vi "test Encoding Error Conditions.vi"(8 "error in":errorcluster, 11 "TestCase in":refnum<class "Encoding and Decoding.lvclass">) -> (0 "error out":errorcluster, 3 "TestCase out":refnum<class "Encoding and Decoding.lvclass">)   [LabVIEW 2020, in "Encoding and Decoding.lvclass"]
uses:
  Encoding and Decoding.lvclass
  Protocol/Implementations/ARINC429/Parameter Definition.ctl
  Encoding and Decoding/Encoding.ctl
  Protocol/Implementations/ARINC429/ARINC429-32bit/32-bit Word.lvclass/32-bit Word.ctl
  4413749d-09be-4b2c-9fd8-42957a21c6ba.vi
  Shared/Encode Parameter and Update Word (32-bit).vi/1445f95d-237d-4fc6-96b9-8992d347f513.vi
  Shared/Encode Parameter and Update Word (32-bit).vi/6b8853f0-8e5d-49e3-9391-4d3f8e5314b0.vi
  Shared/Encode Parameter and Update Word (32-bit).vi/2babc4f4-546e-4d35-846d-a4a1fbac0249.vi
  4413749d-09be-4b2c-9fd8-42957a21c6ba.vi/1980749b-e417-4a21-943a-7c30016504b0.vi
  4413749d-09be-4b2c-9fd8-42957a21c6ba.vi/1f3c3557-5c17-491c-9e18-ef0b55369bc3.vi
  Shared/Encode Parameter and Update Word (32-bit).vi/1445f95d-237d-4fc6-96b9-8992d347f513.vi/22abf0d2-70bd-4b51-a478-b97a2704f7df.vi
  Shared/Encode Parameter and Update Word (32-bit).vi/1445f95d-237d-4fc6-96b9-8992d347f513.vi/c253b733-33bf-43c6-b07a-ea22f5c7a6f3.vi
  Shared/Encode Parameter and Update Word (32-bit).vi/1445f95d-237d-4fc6-96b9-8992d347f513.vi/9377bb8f-44b5-4a8f-87f1-966fd5a9edcc.vi
  Shared/Encode Parameter and Update Word (32-bit).vi/6b8853f0-8e5d-49e3-9391-4d3f8e5314b0.vi/a54b505c-1216-4ef4-8378-3ceda9d188df.vi
  Shared/Encode Parameter and Update Word (32-bit).vi/6b8853f0-8e5d-49e3-9391-4d3f8e5314b0.vi/136dcdcb-2dd3-4a4d-a796-a8f7a3f8e1ac.vi
  4413749d-09be-4b2c-9fd8-42957a21c6ba.vi/1980749b-e417-4a21-943a-7c30016504b0.vi/16a2565b-3c16-407b-a626-9da2a3da432e.vi
  4413749d-09be-4b2c-9fd8-42957a21c6ba.vi/1f3c3557-5c17-491c-9e18-ef0b55369bc3.vi/0a001d06-2809-4638-8d0b-e017d2157007.vi
  Encoding and Decoding/BCD Decode Integer.vi
  Shared/Encode Parameter and Update Word (32-bit).vi/1445f95d-237d-4fc6-96b9-8992d347f513.vi/22abf0d2-70bd-4b51-a478-b97a2704f7df.vi/9d450a76-0fc9-4555-8e71-4c202274969f.vi
  Shared/Encode Parameter and Update Word (32-bit).vi/1445f95d-237d-4fc6-96b9-8992d347f513.vi/c253b733-33bf-43c6-b07a-ea22f5c7a6f3.vi/9d450a76-0fc9-4555-8e71-4c202274969f.vi
  Shared/Encode Parameter and Update Word (32-bit).vi/6b8853f0-8e5d-49e3-9391-4d3f8e5314b0.vi/a54b505c-1216-4ef4-8378-3ceda9d188df.vi/a7fcce85-1f75-4572-aeaa-ddfd463a7c5f.vi
  Encoding and Decoding/BCD Decode Integer.vi/9a65bfc0-0d77-4ef3-ab58-63df1e1caa90.vi
  Protocol/Implementations/ARINC429/ARINC429-32bit/32-bit Word.lvclass
  <vilib>/addons/_JKI Toolkits/VI Tester/TestCase.llb/TestCase.lvclass
  Encoding and Decoding/Encoding and Decoding.lvlib
  Protocol/Implementations/ARINC429/ARINC 429.lvclass
  C:/Program Files (x86)/National Instruments/LabVIEW 2020/vi.lib/addons/_JKI Toolkits/VI Tester/TestCase.llb/TestCase.lvclass
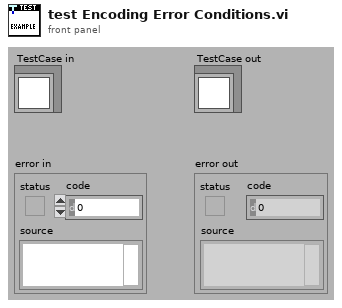
[diagram p1: front panel]
types:
  T1 = typedef "ARINC 429.lvclass/Parameter Definition.ctl" = cluster{"start index":i32, "size":i32, "encoding":T2, "signed":bool, "scale multiplier":dbl, "scale offset":dbl}
  T2 = typedef "Encoding and Decoding.lvlib/Encoding.ctl" = enum16{"BNR", "BCD", "Discrete"}
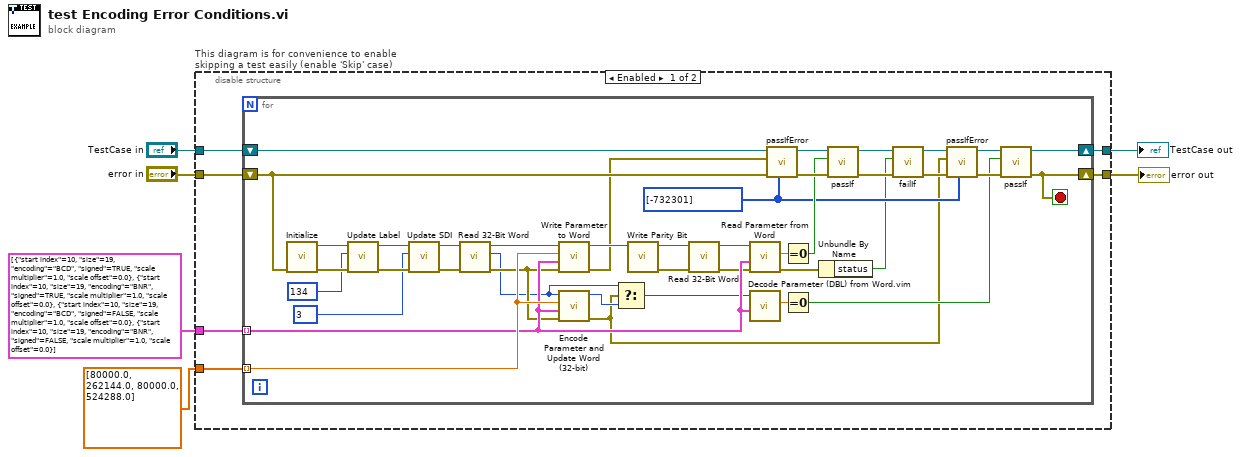
[diagram p0: block diagram]
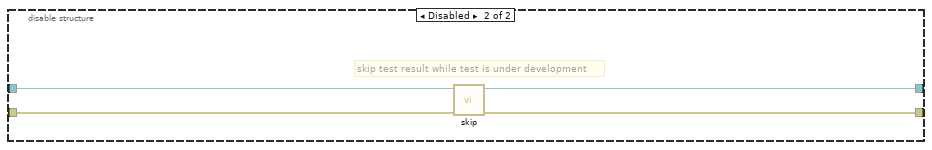
[diagram p2: hidden frame]
diagram:
  n1 = disable-structure "This diagram is for convenience to enable skipping a test easily (enable 'Skip' case)" shown="Enabled" {
    disable-tunnel: "TestCase in" -> [w12 w57]
    disable-tunnel: [w11 w55] -> w3
    disable-tunnel: [w10 w56] -> w5
    disable-tunnel: "error in" -> [w7 w54]
    disable-tunnel: T1[] [{"start index"=10, "size"=19, "encoding"=enum."BCD", "signed"=TRUE, "scale multiplier"=1.0, "scale offset"=0.0}, {"start index"=10, "size"=19, "encoding"=enum."BNR", "signed"=TRUE, "scale multiplier"=1.0, "scale offset"=0.0}, {"start index"=10, "size"=19, "encoding"=enum."BCD", "signed"=FALSE, "scale multiplier"=1.0, "scale offset"=0.0}, {"start index"=10, "size"=19, "encoding"=enum."BNR", "signed"=FALSE, "scale multiplier"=1.0, "scale offset"=0.0}] -> [w8 _]
    disable-tunnel: dbl[] [80000.0, 262144.0, 80000.0, 524288.0] -> [w9 _]
    frame Enabled {
      n2 = for {
        tunnel: w9 -> [w33] mode=indexing
        tunnel: w8 -> [w32] mode=indexing
        shift-right: [w34] -> w11
        shift-left: w12 -> [w40]
        shift-right: [w13] -> w10
        shift-left: w7 -> [w30]
        stop <- w13 stop-if-true
        w27 = i32[] [-732301] ("passing error codes (default = any error code)")
        n3 = call "Initialize.vi"("error in"=w30) -> ("error out"=w49:errorcluster, "ARINC 429 (32-bit word)"=w44:refnum<class "32-bit Word.lvclass">)  [unwired: 9 in]
        n4 = call-dynamic "Update Label.vi"("error in"=w49, "label value"=u8 134 ("label value 2"), "32-bit word in"=w44) -> ("error out"=w50:errorcluster, "32-bit word out"=w47:refnum<class "32-bit Word.lvclass">)  [unwired: 7 in]
        n5 = call-dynamic "Update SDI.vi"("error in"=w50, "SDI value"=u8 3 ("SDI value 2"), "32-bit Word in"=w47) -> ("error out"=w38:errorcluster, "32-bit Word out"=w39:refnum<class "32-bit Word.lvclass">)  [unwired: 7 in]
        n6 = call "Read 32-Bit Word.vi"("error in (no error)"=w38, "32-bit Word in"=w39) -> ("error out"=w26:errorcluster, "32-bit word"=w15:u32, "32-bit Word out"=w37:refnum<class "32-bit Word.lvclass">)  [unwired: 7 in]
        n7 = call-dynamic "Write Parameter to Word.vi"("error in"=w26, "parameter definition"=w32, "data"=w33, "32-bit Word in"=w37) -> ("error out"=w24:errorcluster, "32-bit Word out"=w52:refnum<class "32-bit Word.lvclass">)  [unwired: 6 in]
        n8 = call "Encode Parameter and Update Word (32-bit).vi"("error in"=w26, "parameter definition"=w32, "parameter value"=w33, "word in"=w15) -> ("error out"=w16:errorcluster, "word out"=w17:u32)  [unwired: 6 in]
        n9 = Select(t=w15, s=w16, f=w17) -> (s? t:f=w14:u32)
        n10 = call-dynamic "Write Parity Bit.vi"("32-bit word in"=w52) -> ("error out"=w51:errorcluster, "32-bit word out"=w48:refnum<class "32-bit Word.lvclass">)  [unwired: 9 in]
        n11 = call "Read 32-Bit Word.vi"("error in (no error)"=w51, "32-bit Word in"=w48) -> ("error out"=w25:errorcluster, "32-bit Word out"=w53:refnum<class "32-bit Word.lvclass">)  [unwired: 7 in, 1 out]
        n12 = call-dynamic "Read Parameter from Word.vi"("error in"=w25, "parameter definition"=w32, "32-bit Word in"=w53) -> ("error out"=w19:errorcluster, "parameter value"=w41:dbl)  [unwired: 6 in, 1 out]
        n13 = call "Decode Parameter (DBL) from Word.vim"("parameter definition"=w32, "32-bit word in"=w14) -> ("parameter value"=w29:dbl)  [unwired: 7 in, 2 out]
        n14 = call-dynamic "passIfError.vi"("passing error codes (default = any error code)"=w27, "error in (no error)"=w30, "error"=w24, "TestCase in"=w40) -> ("error out"=w42:errorcluster, "TestCase out"=w43:refnum<class "Encoding and Decoding.lvclass">)  [unwired: 6 in]
        n15 = Equal To 0?(x=w41) -> (x = 0?=w31:bool)
        n16 = Equal To 0?(x=w29) -> (x = 0?=w28:bool)
        n17 = Unbundle By Name(w19) -> ("status"=w18:bool)
        n18 = call-dynamic "passIf.vi"("error in (no error)"=w42, "pass"=w31, "TestCase in"=w43) -> ("error out"=w22:errorcluster, "TestCase out"=w23:refnum<class "Encoding and Decoding.lvclass">)  [unwired: 7 in]
        n19 = call-dynamic "failIf.vi"("error in (no error)"=w22, "fail"=w18, "TestCase in"=w23) -> ("error out"=w20:errorcluster, "TestCase out"=w21:refnum<class "Encoding and Decoding.lvclass">)  [unwired: 7 in]
        n20 = call-dynamic "passIfError.vi"("passing error codes (default = any error code)"=w27, "error in (no error)"=w20, "error"=w16, "TestCase in"=w21) -> ("error out"=w36:errorcluster, "TestCase out"=w35:refnum<class "Encoding and Decoding.lvclass">)  [unwired: 6 in]
        n21 = call-dynamic "passIf.vi"("error in (no error)"=w36, "pass"=w28, "TestCase in"=w35) -> ("error out"=w13:errorcluster, "TestCase out"=w34:refnum<class "Encoding and Decoding.lvclass">)  [unwired: 7 in]
      }
    }
    frame Disabled {
      # "skip test result while test is under development"
      n22 = call <vilib>:"skip.vi"("error in (no error)"=w54, "TestCase in"=w57) -> ("error out"=w56:errorcluster, "TestCase out"=w55:refnum<class "Encoding and Decoding.lvclass">)  [unwired: 8 in]
    }
  }
  "error out" <- w5
  "TestCase out" <- w3
